vi "Get Database Connection.vi"() -> (0 "Database Settings":T1={"Data Source Name"="HANSPH_LAPTOP\\SQLEXPRESS", "Database Name"="MEASUREMENTS", "User Name"="sa", "Password"=""}, 1 "Database  Connection String":string)   [LabVIEW 2019]
uses:
  <vilib>/Utility/config.llb/Read Key (String).vi
  <vilib>/Utility/config.llb/NI_LVConfig.lvlib
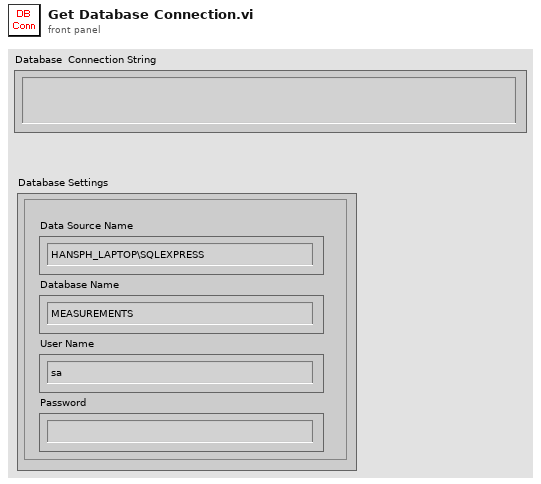
[diagram p1: front panel]
types:
  T1 = cluster{"Data Source Name":string, "Database Name":string, "User Name":string, "Password":string}
  T2 = typedef "NI_LVConfig.lvlib/Config Data RefNum.ctl" = refnum<k1>
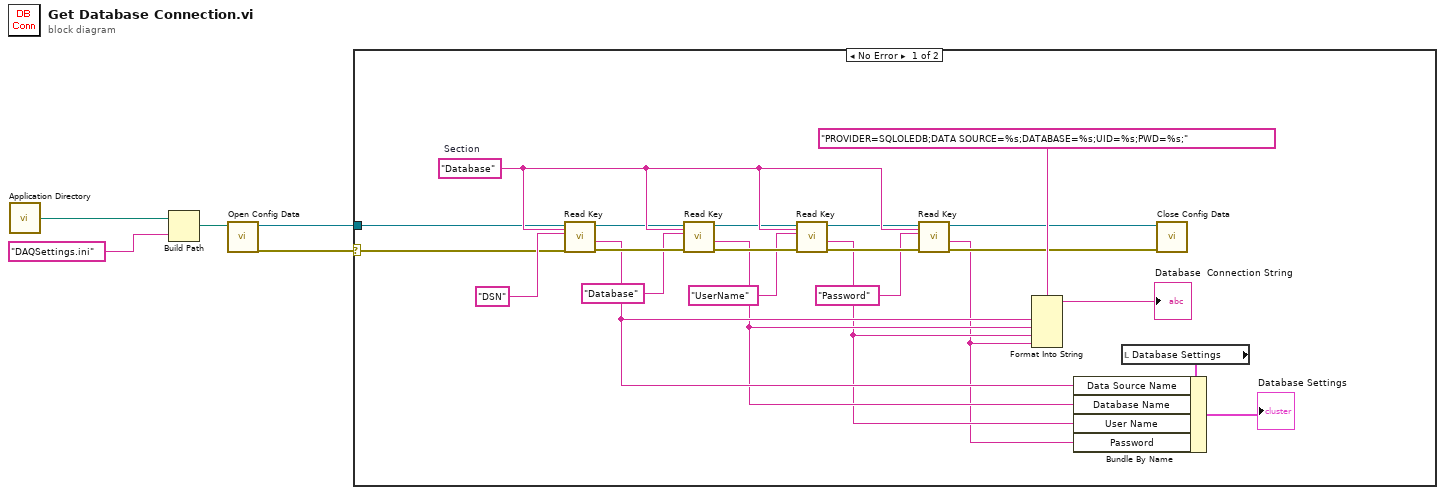
[diagram p0: block diagram]
diagram:
  n1 = call <vilib>:"Application Directory.vi"() -> ("Application Directory"=w5:path)
  n2 = Build Path(base path=w5, name or relative path="DAQSettings.ini") -> (appended path=w3:path)
  n3 = call <vilib>:"Open Config Data.vi"("configuration file path"=w3) -> ("error out"=w1:errorcluster, "refnum"=w2:T2)  [unwired: 8 in, 1 out]
  n4 = case shown="No Error" w1 {
    selector: w1 -> [w13 _]
    tunnel: w2 -> [w14 _]
    frame No Error {
      w28 = "Database"  # Section
      n5 = call-poly <vilib>:"Read Key.vi"("section"=w28, "error in (no error)"=w13, "key"="DSN", "refnum"=w14) -> ("error out"=w19:errorcluster, "value"=w11:string, "refnum out"=w20:T2)  [unwired: 4 in, 1 out]
      n6 = call-poly <vilib>:"Read Key.vi"("section"=w28, "error in (no error)"=w19, "key"="Database", "refnum"=w20) -> ("error out"=w25:errorcluster, "value"=w10:string, "refnum out"=w24:T2)  [unwired: 4 in, 1 out]
      n7 = call-poly <vilib>:"Read Key.vi"("section"=w28, "error in (no error)"=w25, "key"="UserName", "refnum"=w24) -> ("error out"=w27:errorcluster, "value"=w9:string, "refnum out"=w26:T2)  [unwired: 4 in, 1 out]
      n8 = call-poly <vilib>:"Read Key.vi"("section"=w28, "error in (no error)"=w27, "key"="Password", "refnum"=w26) -> ("error out"=w15:errorcluster, "value"=w8:string, "refnum out"=w16:T2)  [unwired: 4 in, 1 out]
      n9 = Format Into String(format string="PROVIDER=SQLOLEDB;DATA SOURCE=%s;DATABASE=%s;UID=%s;PWD=%s;", w11, w10, w9, w8) -> (resulting string=→"Database  Connection String":string)  [unwired: 2 in, 1 out]
      n10 = local read "Database Settings"() -> (w6:T1)
      n11 = Bundle By Name(cluster=w6, "Data Source Name"=w11, "Database Name"=w10, "User Name"=w9, "Password"=w8) -> (→"Database Settings":T1)
      n12 = call <vilib>:"Close Config Data.vi"("error in (no error)"=w15, "refnum"=w16) -> ()  [unwired: 8 in, 2 out]
    }
    frame Error {
    }
  }
